vi "ModifyMyAttribute.vi"(0 "reference in":refnum<class "MyG#SubClass.lvclass">, 2 "increment":dbl, 5 "error in (no error)":errorcluster) -> (14 "reference out":refnum<class "MyG#SubClass.lvclass">, 19 "error out":errorcluster)   [LabVIEW 2020, in "MyG#SubClass.lvclass"]
uses:
  MyG#SubClass.lvclass
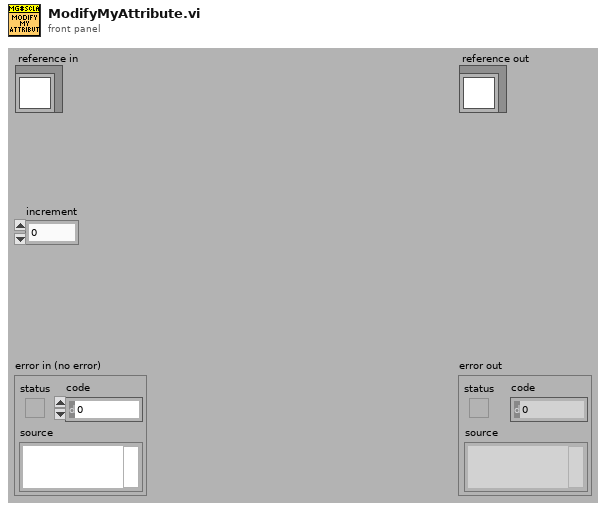
[diagram p1: front panel]
types:
  T1 = typedef "MyG#SubClass.lvclass/ObjectAttributesRef.ctl" = refnum<data-value>
  T2 = typedef "MyG#SubClass.lvclass/ObjectAttributes.ctl" = cluster{"MySubAttribute":dbl}
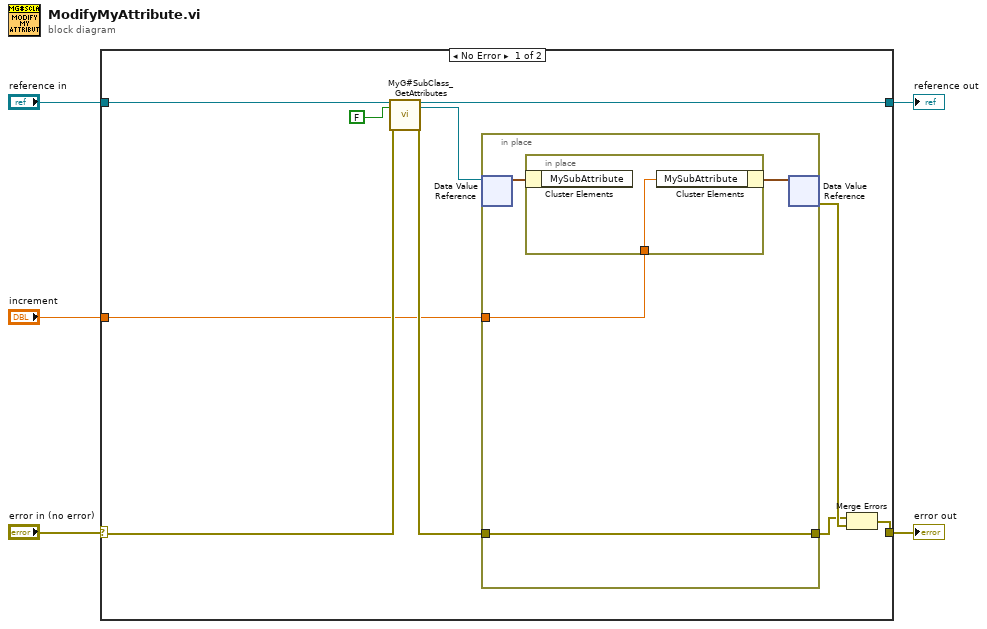
[diagram p0: block diagram]
diagram:
  n1 = case shown="No Error" "error in (no error)" {
    selector: "error in (no error)" -> [w10 w22]
    tunnel: [w15 w22] -> w4
    tunnel: [w8 w21] -> w2
    tunnel: "reference in" -> [w12 w21]
    tunnel: "increment" -> [w6 _]
    frame No Error {
      n2 = call "MyG#SubClass_GetAttributes.vi"("reference in"=w12, "return data? (T)"=FALSE, "error in (no error)"=w10) -> ("reference out"=w8:refnum<class "MyG#SubClass.lvclass">, "attributes ref"=w7:T1, "error out"=w9:errorcluster)  [unwired: 13 in, 1 out]
      n3 = in-place {
        in-place-border: w9 -> [w17]
        in-place-border: [w17] -> w13
        in-place-border: w6 -> [w16]
        n4 = in-place-dvr #1(w7) -> (w18:T2)  [unwired: 1 out]
        n5 = in-place {
          in-place-border: w16 -> [w20]
          n6 = in-place-cluster #2(w18) -> ()  [unwired: 1 out]
          n7 = in-place-cluster #2("MySubAttribute"=w20) -> (w19:T2)
        }
        n8 = in-place-dvr #1(w19) -> (w14:errorcluster)  [unwired: 1 out]
      }
      n9 = Merge Errors(w13, w14) -> (w15:errorcluster)
    }
    frame Error {
    }
  }
  "error out" <- w4
  "reference out" <- w2
